vi "ConfigParams - Parse - CAN.vi"(8 "error in (no error)":errorcluster, 11 "Ethernet in":refnum<class "ENET_BS1201.lvclass">) -> (0 "error out":errorcluster, 1 "WritePeriod_ms":i32=5, 2 "BoxID":i32=54321, 3 "Ethernet out":refnum<class "ENET_BS1201.lvclass">)   [LabVIEW 2021, in "BS120x Driver.lvlib" / "ENET_BS1201.lvclass"]
uses:
  ENET_BS1201.lvclass
panel:
  # "[CAN]\nInterfaceIndex = 0\nBoxID = 1\nBaudRate = 1000000\nRcvQueueSize = 64\nWritePeriod_ms = 5"
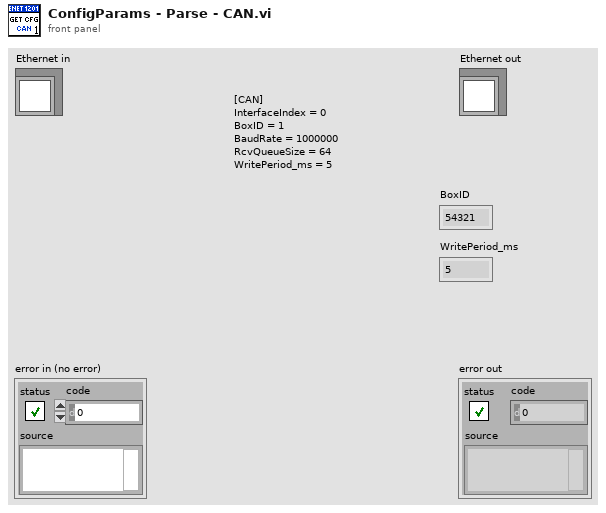
[diagram p1: front panel]
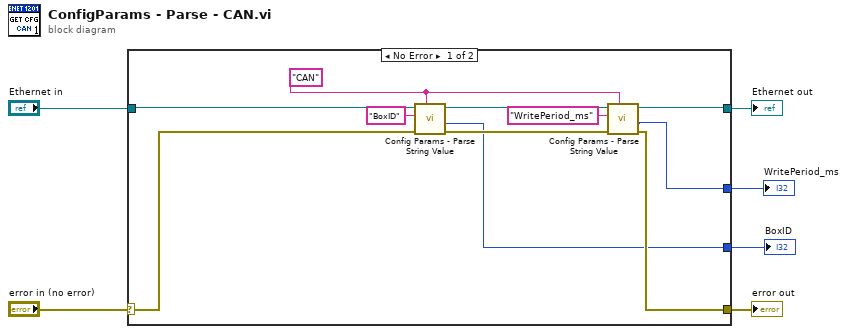
[diagram p0: block diagram]
diagram:
  n1 = case shown="No Error" "error in (no error)" {
    selector: "error in (no error)" -> [w7 w19]
    tunnel: [w11 w19] -> w5
    tunnel: [w12 w18] -> w3
    tunnel: "Ethernet in" -> [w8 w18]
    tunnel: [w10 _] -> w2
    tunnel: [w9 _] -> w1
    frame No Error {
      w14 = "CAN" ("Section")
      n2 = call-dynamic "Config Params - Parse String Value.vi"("Section"=w14, "error in (no error)"=w7, "Key"="BoxID", "Ethernet in"=w8) -> ("error out"=w15:errorcluster, "Value (int)"=w10:i32, "Ethernet out"=w16:refnum<class "ENET_BS1201.lvclass">)  [unwired: 1 in, 4 out]
      n3 = call-dynamic "Config Params - Parse String Value.vi"("Section"=w14, "error in (no error)"=w15, "Key"="WritePeriod_ms", "Ethernet in"=w16) -> ("error out"=w11:errorcluster, "Value (int)"=w9:i32, "Ethernet out"=w12:refnum<class "ENET_BS1201.lvclass">)  [unwired: 1 in, 4 out]
    }
    frame Error {
    }
  }
  "error out" <- w5
  "Ethernet out" <- w3
  "BoxID" <- w2
  "WritePeriod_ms" <- w1
